vi "Query.vi"() -> ()   [LabVIEW 2017]
panel:
  in  "Close":bool
  out "Results":string
  in  "search":bool
  in  "AndOr2":enum16{"And", "Or"}(ring)=enum."Or"
  in  "AndOr1":enum16{"And", "Or"}(ring)=enum."Or"
  in  "Answer 3":string(combo)
  in  "Question 3":string(combo)
  in  "Answer 2":string(combo)
  in  "Question 2":string(combo)
  in  "Answer 1":string(combo)
  in  "Question 1":string(combo)
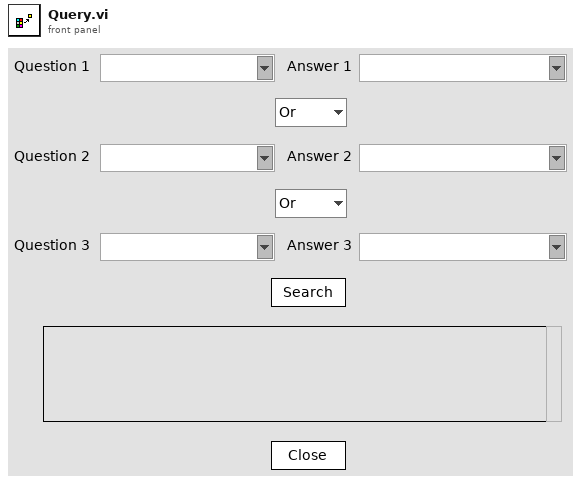
[diagram p1: front panel]
types:
  T1 = cluster{"question":string, "Answers":cluster{"answer":string, "Teams":i32[]}[]}[]
  T2 = cluster{"question":string, "Answers":cluster{"answer":string, "Teams":i32[]}[]}
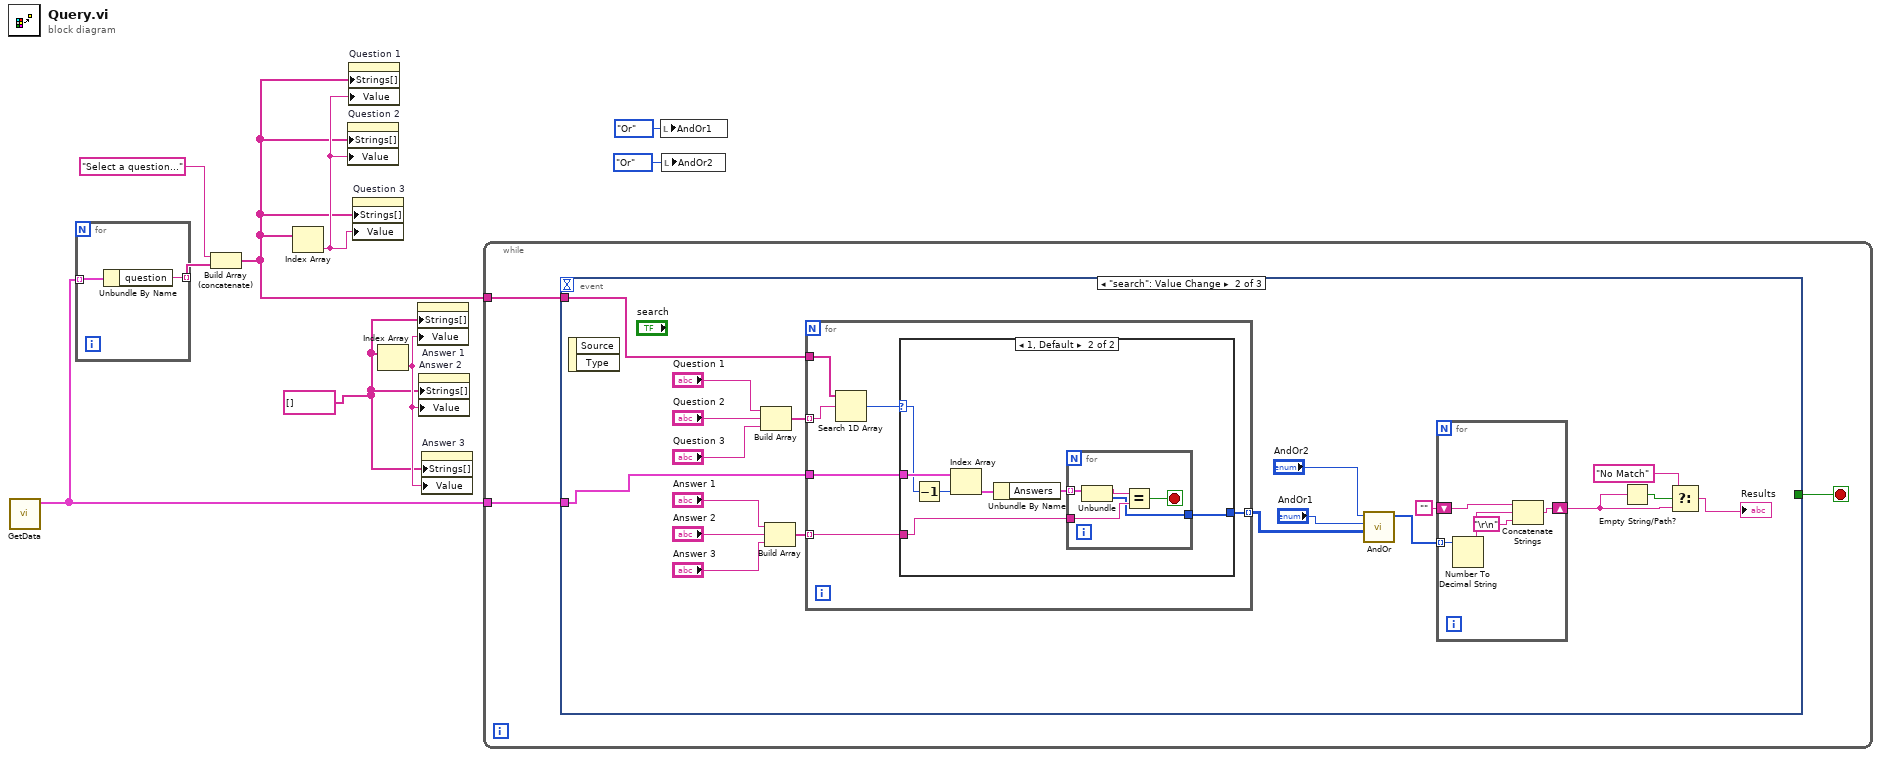
[diagram p0: block diagram]
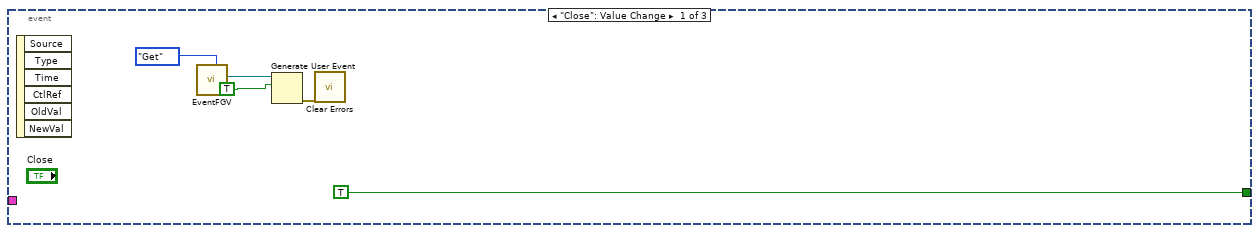
[diagram p2: hidden frame]
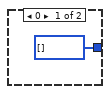
[diagram p3: hidden frame]
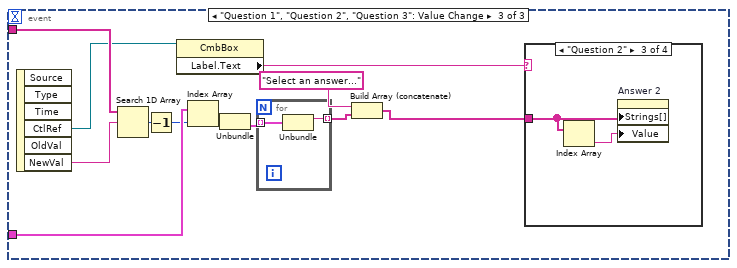
[diagram p4: hidden frame]
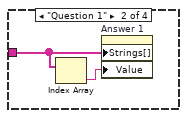
[diagram p6: hidden frame]
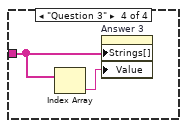
[diagram p7: hidden frame]
diagram:
  w3 = string[] [] ("appended array")
  n1 = call "GetData.vi"() -> ("Array"=w9:T1)  [unwired: 11 in]
  n2 = for {
    tunnel: w9 -> [w11] mode=indexing
    tunnel: [w10] -> w8 mode=indexing
    n3 = Unbundle By Name(w11) -> ("question"=w10:string)
  }
  n4 = Build Array (concatenate)("Select a question...", w8) -> (w6:string[])
  n5 = Index Array(array=w6) -> (element=w7:string)  [unwired: 1 in]
  n6 = property on="Question 2" class="CmbBox"("Strings[]"=w6, "Value"=w7) -> ()  [unwired: 2 in, 2 out]
  n7 = property on="Question 1" class="CmbBox"("Strings[]"=w6, "Value"=w7) -> ()  [unwired: 2 in, 2 out]
  n8 = property on="Question 3" class="CmbBox"("Strings[]"=w6, "Value"=w7) -> ()  [unwired: 2 in, 2 out]
  n9 = Index Array(array=w3) -> (element=w4:string)  [unwired: 1 in]
  n10 = property on="Answer 1" class="CmbBox"("Strings[]"=w3, "Value"=w4) -> ()  [unwired: 2 in, 2 out]
  n11 = property on="Answer 2" class="CmbBox"("Strings[]"=w3, "Value"=w4) -> ()  [unwired: 2 in, 2 out]
  n12 = property on="Answer 3" class="CmbBox"("Strings[]"=w3, "Value"=w4) -> ()  [unwired: 2 in, 2 out]
  n13 = while {
    tunnel: w9 -> [w13]
    tunnel: w6 -> [w12]
    stop <- w14 stop-if-true
    n14 = event shown="[1] \"search\": Value Change" {
      selector: _ -> [_ _ _]
      dyn-events: _ -> [_ _ _]
      timeout: _ -> [_ _ _]
      tunnel: [TRUE _ _] -> w14
      tunnel: w13 -> [_ w30 w71]
      tunnel: w12 -> [_ w29 w73]
      event "Close": Value Change {
        n15 = event-data() -> ()  [unwired: 1 in, 6 out]
        n16 = call "EventFGV.vi"("Action"=enum16{"Set", "Get"}."Get") -> ("user event out"=w18:refnum<user-event>)  [unwired: 10 in]
        n17 = Generate User Event(user event=w18, event data cluster=TRUE ("event data")) -> (error out=w15:errorcluster)  [unwired: 2 in, 1 out]
        n18 = call <vilib>:"Clear Errors.vi"("error in (no error)"=w15) -> ()  [unwired: 5 in, 2 out]
      }
      event "search": Value Change {
        n19 = event-data() -> ()  [unwired: 1 in, 2 out]
        n20 = Build Array("Question 1", "Question 2", "Question 3") -> (w32:string[])
        n21 = Build Array("Answer 1", "Answer 2", "Answer 3") -> (w31:string[])
        n22 = for {
          tunnel: w32 -> [w44] mode=indexing
          tunnel: w31 -> [w40] mode=indexing
          tunnel: w30 -> [w41]
          tunnel: w29 -> [w43]
          tunnel: [w39] -> w28 mode=indexing
          n23 = Search 1D Array(1D array=w43, element=w44) -> (index of element=w42:i32)  [unwired: 1 in]
          n24 = case shown="1, Default" w42 {
            selector: w42 -> [_ w51]
            tunnel: w41 -> [_ w52]
            tunnel: w40 -> [_ w47]
            tunnel: [i32[] [] ("Teams") w46] -> w39
            frame 0 {
            }
            frame 1, Default {
              n25 = Decrement(x=w51) -> (x-1=w50:i32)
              n26 = Index Array(array=w52, index=w50) -> (element=w49:T2)
              n27 = Unbundle By Name(w49) -> ("Answers"=w48:cluster{"answer":string, "Teams":i32[]}[])
              n28 = for {
                tunnel: w48 -> [w57] mode=indexing
                tunnel: w47 -> [w56]
                tunnel: [w53] -> w46
                stop <- w54 stop-if-true
                n29 = Unbundle(w57) -> ("answer"=w55:string, "Teams"=w53:i32[])
                n30 = Equal?(x=w55, y=w56) -> (x = y?=w54:bool)
              }
            }
          }
        }
        n31 = call "AndOr.vi"("Teams in"=w28, "AndOr1"="AndOr1", "AndOr2"="AndOr2") -> ("Teams out"=w27:i32[])  [unwired: 8 in]
        n32 = for {
          tunnel: w27 -> [w60] mode=indexing
          shift-right: [w62] -> w24
          shift-left: "" -> [w61]
          n33 = Number To Decimal String(number=w60) -> (decimal integer string=w59:string)  [unwired: 1 in]
          n34 = Concatenate Strings(w61, w59, "\r\n") -> (w62:string)
        }
        n35 = Empty String/Path?(string/path=w24) -> (empty?=w25:bool)
        n36 = Select(t="No Match", s=w25, f=w24) -> (s? t:f=→"Results":string)
      }
      event "Question 1", "Question 2", "Question 3": Value Change {
        n37 = event-data() -> ("CtlRef"=w69:refnum<vi>, "NewVal"=w74:string)  [unwired: 1 in, 4 out]
        n38 = Search 1D Array(1D array=w73, element=w74) -> (index of element=w72:i32)  [unwired: 1 in]
        n39 = Decrement(x=w72) -> (x-1=w66:i32)
        n40 = property class="CmbBox"(reference=w69) -> ("Label.Text"=w68:string)  [unwired: 1 in, 2 out]
        n41 = Index Array(array=w71, index=w66) -> (element=w70:T2)
        n42 = Unbundle(w70) -> ("Answers"=w67:cluster{"answer":string, "Teams":i32[]}[])  [unwired: 1 out]
        n43 = for {
          tunnel: w67 -> [w82] mode=indexing
          tunnel: [w81] -> w64 mode=indexing
          n44 = Unbundle(w82) -> ("answer"=w81:string)  [unwired: 1 out]
        }
        n45 = Build Array (concatenate)("Select an answer...", w64) -> (w63:string[])
        n46 = case shown="\"Question 2\"" w68 {
          tunnel: w63 -> [_ w75 w77 w80]
          frame "False", Default {
          }
          frame "Question 1" {
            n47 = Index Array(array=w75) -> (element=w76:string)  [unwired: 1 in]
            n48 = property on="Answer 1" class="CmbBox"("Strings[]"=w75, "Value"=w76) -> ()  [unwired: 2 in, 2 out]
          }
          frame "Question 2" {
            n49 = Index Array(array=w77) -> (element=w78:string)  [unwired: 1 in]
            n50 = property on="Answer 2" class="CmbBox"("Strings[]"=w77, "Value"=w78) -> ()  [unwired: 2 in, 2 out]
          }
          frame "Question 3" {
            n51 = Index Array(array=w80) -> (element=w79:string)  [unwired: 1 in]
            n52 = property on="Answer 3" class="CmbBox"("Strings[]"=w80, "Value"=w79) -> ()  [unwired: 2 in, 2 out]
          }
        }
      }
    }
  }
  n53 = local write "AndOr1"(enum16{"And", "Or"}."Or" ("AndOr2")) -> ()
  n54 = local write "AndOr2"(enum16{"And", "Or"}."Or" ("AndOr2")) -> ()
